vi "RotatePointstoY.vi"(0 "x matrix":dbl[][](array[numeric]) format="%.2f", 1 "y matrix":dbl[][](array[numeric]) format="%.2f", 2 "z matrix":dbl[][](array[numeric]) format="%.2f", 3 "x matrix 1D":dbl[](array[numeric]) format="%.2f", 4 "y matrix 1D":dbl[](array[numeric]) format="%.2f", 5 "z matrix 1D":dbl[](array[numeric]) format="%.2f", 6 "P":cluster{"x":dbl, "y":dbl, "z":dbl} {"z" format="%.2f"; "y" format="%.2f"; "x" format="%.2f"}) -> (12 "transfrom matrix":dbl[][](array[numeric]) format="%.2f", 14 "x matrix":dbl[][](array[numeric]) format="%.2f", 15 "y matrix":dbl[][](array[numeric]) format="%.2f", 16 "z matrix":dbl[][](array[numeric]) format="%.2f", 17 "x matrix1D":dbl[](array[numeric]) format="%.2f", 18 "y matrix 1D":dbl[](array[numeric]) format="%.2f", 19 "z matrix 1D":dbl[](array[numeric]) format="%.2f")   [LabVIEW 2022 SP3]
uses:
  <vilib>/Analysis/baseanly.llb/A x Vector.vi
  <vilib>/Analysis/NI_AALBase.lvlib
panel:
  # "output side"
  # "Input side"
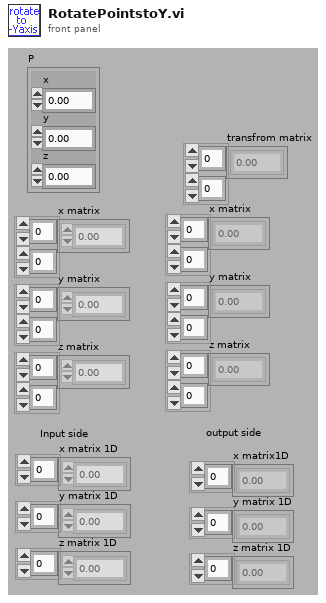
[diagram p1: front panel]
types:
  T1 = cluster{"A x Vector[0]":dbl, "A x Vector[1]":dbl, "A x Vector[2]":dbl}
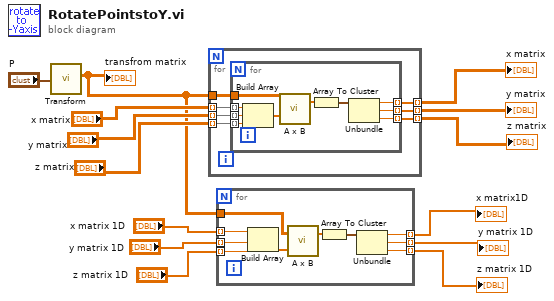
[diagram p0: block diagram]
diagram:
  n1 = call "Transform.vi"("P"="P") -> ("transfrom matrix"=w4:dbl[][])  [unwired: 4 out]
  "transfrom matrix" <- w4
  n2 = for {
    tunnel: "x matrix" -> [w21] mode=indexing
    tunnel: "y matrix" -> [w20] mode=indexing
    tunnel: "z matrix" -> [w19] mode=indexing
    tunnel: [w18] -> w11 mode=indexing
    tunnel: [w17] -> w12 mode=indexing
    tunnel: [w16] -> w13 mode=indexing
    tunnel: w4 -> [w15]
    n3 = for {
      tunnel: [w30] -> w18 mode=indexing
      tunnel: [w29] -> w17 mode=indexing
      tunnel: [w28] -> w16 mode=indexing
      tunnel: w21 -> [w27] mode=indexing
      tunnel: w20 -> [w26] mode=indexing
      tunnel: w19 -> [w25] mode=indexing
      tunnel: w15 -> [w22]
      n4 = Build Array(w27, w26, w25) -> (w23:dbl[])
      n5 = call-poly <vilib>:"A x B.vi"("Vector"=w23, "A"=w22) -> ("A x Vector"=w24:dbl[])  [unwired: 1 out]
      n6 = Array To Cluster(array=w24) -> (cluster=w31:T1)
      n7 = Unbundle(w31) -> ("A x Vector[0]"=w30:dbl, "A x Vector[1]"=w29:dbl, "A x Vector[2]"=w28:dbl)
    }
  }
  "z matrix" <- w13
  "y matrix" <- w12
  "x matrix" <- w11
  n8 = for {
    tunnel: [w40] -> w3 mode=indexing
    tunnel: [w39] -> w2 mode=indexing
    tunnel: [w38] -> w1 mode=indexing
    tunnel: "x matrix 1D" -> [w36] mode=indexing
    tunnel: "y matrix 1D" -> [w35] mode=indexing
    tunnel: "z matrix 1D" -> [w34] mode=indexing
    tunnel: w4 -> [w32]
    n9 = Build Array(w36, w35, w34) -> (w33:dbl[])
    n10 = call-poly <vilib>:"A x B.vi"("Vector"=w33, "A"=w32) -> ("A x Vector"=w37:dbl[])  [unwired: 1 out]
    n11 = Array To Cluster(array=w37) -> (cluster=w41:T1)
    n12 = Unbundle(w41) -> ("A x Vector[0]"=w40:dbl, "A x Vector[1]"=w39:dbl, "A x Vector[2]"=w38:dbl)
  }
  "z matrix 1D" <- w1
  "y matrix 1D" <- w2
  "x matrix1D" <- w3
